vi "Create Arm.vi"(6 "New Object":refnum<vi>, 7 "Arm Cluster":T1) -> (0 "EJC":refnum<vi>, 2 "New Object":refnum<vi>, 3 "SJC":refnum<vi>, 4 "reference out":refnum<vi>)   [LabVIEW 2010]
uses:
  <vilib>/picture/3D Picture Control/NI_3D Picture Control.lvlib
panel:
  out "3D Picture":refnum<vi>(3d-picture)
  out "Forearm":refnum<vi>
  out "Humerus":refnum<vi>
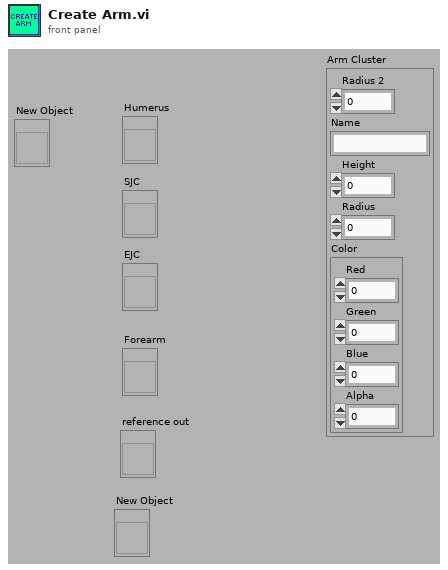
[diagram p1: front panel]
types:
  T1 = cluster{"Radius 2":sgl, "Name":string, "Height":sgl, "Radius":sgl, "Color":cluster{"Red":sgl, "Green":sgl, "Blue":sgl, "Alpha":sgl}}
  T2 = cluster{"Red":sgl, "Green":sgl, "Blue":sgl, "Alpha":sgl}
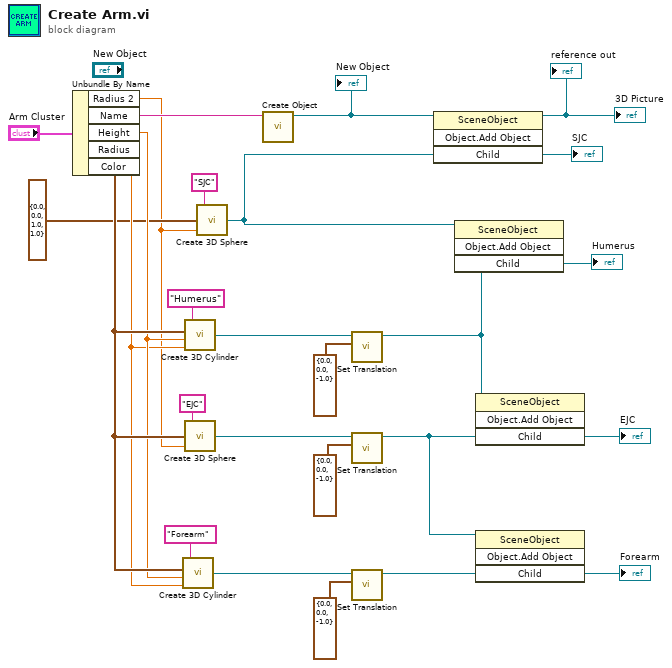
[diagram p0: block diagram]
diagram:
  n1 = Unbundle By Name("Arm Cluster") -> ("Radius 2"=w1:sgl, "Name"=w3:string, "Height"=w20:sgl, "Radius"=w19:sgl, "Color"=w21:T2)
  n2 = call "Create 3D Cylinder.vi"("Radius"=w19, "Height"=w20, "Color"=w21, "Name"="Forearm") -> ("Scene:New Object"=w10:refnum<vi>)
  n3 = call "Create 3D Cylinder.vi"("Radius"=w19, "Height"=w20, "Color"=w21, "Name"="Humerus") -> ("Scene:New Object"=w15:refnum<vi>)
  n4 = call "Create 3D Sphere.vi"("Radius"=w1, "Color"=w21, "Name"="EJC") -> ("Scene:New Object"=w13:refnum<vi>)
  n5 = call "Create 3D Sphere.vi"("Radius"=w1, "Color"=T2 {"Red"=0.0, "Green"=0.0, "Blue"=1.0, "Alpha"=1.0}, "Name"="SJC") -> ("Scene:New Object"=w4:refnum<vi>)
  n6 = call <vilib>:"Create Object.vi"("Name"=w3) -> ("Scene:New Object"=w2:refnum<vi>)  [unwired: 9 in, 1 out]
  "New Object" <- w2
  n7 = call <vilib>:"Set Translation.vi"("Translation"=cluster{"X":sgl, "Y":sgl, "Z":sgl} {"X"=0.0, "Y"=0.0, "Z"=-1.0} ("Axis"), "Scene Object"=w15) -> ("Translated Object"=w7:refnum<vi>)  [unwired: 8 in, 1 out]
  n8 = call <vilib>:"Set Translation.vi"("Translation"=cluster{"X":sgl, "Y":sgl, "Z":sgl} {"X"=0.0, "Y"=0.0, "Z"=-1.0} ("Axis"), "Scene Object"=w13) -> ("Translated Object"=w8:refnum<vi>)  [unwired: 8 in, 1 out]
  n9 = call <vilib>:"Set Translation.vi"("Translation"=cluster{"X":sgl, "Y":sgl, "Z":sgl} {"X"=0.0, "Y"=0.0, "Z"=-1.0} ("Axis"), "Scene Object"=w10) -> ("Translated Object"=w9:refnum<vi>)  [unwired: 8 in, 1 out]
  n10 = invoke class="SceneObject" method="Object.Add Object"(reference=w2, "Child"=w4) -> (reference out=→"3D Picture" →"reference out":refnum<vi>, "Child"=→"SJC":refnum<vi>)  [unwired: 2 in, 2 out]
  n11 = invoke class="SceneObject" method="Object.Add Object"(reference=w4, "Child"=w7) -> ("Child"=→"Humerus":refnum<vi>)  [unwired: 2 in, 3 out]
  n12 = invoke class="SceneObject" method="Object.Add Object"(reference=w7, "Child"=w8) -> ("Child"=→"EJC":refnum<vi>)  [unwired: 2 in, 3 out]
  n13 = invoke class="SceneObject" method="Object.Add Object"(reference=w8, "Child"=w9) -> ("Child"=→"Forearm":refnum<vi>)  [unwired: 2 in, 3 out]
